vi "pressure_calcStress.vi"(9 "Pressure":dbl format="%#_13g", 10 "Angle":dbl, 11 "main_FGV_data":T1) -> (1 "PressCircOval":dbl, 2 "PressCirc":dbl, 3 "PressLong":dbl)   [LabVIEW 2016]
uses:
  MainFGV/main_FGV_data.ctl
  MainFGV/pipe_properties.ctl
  StressCalculations/point_data.ctl
  Ovalization/ovalization_data.ctl
  StressDist/StressDist_data.ctl
  StressDist/StressDist_single_data.ctl
  StressDist/Peirce/peirce_data.ctl
  pressure_data.ctl
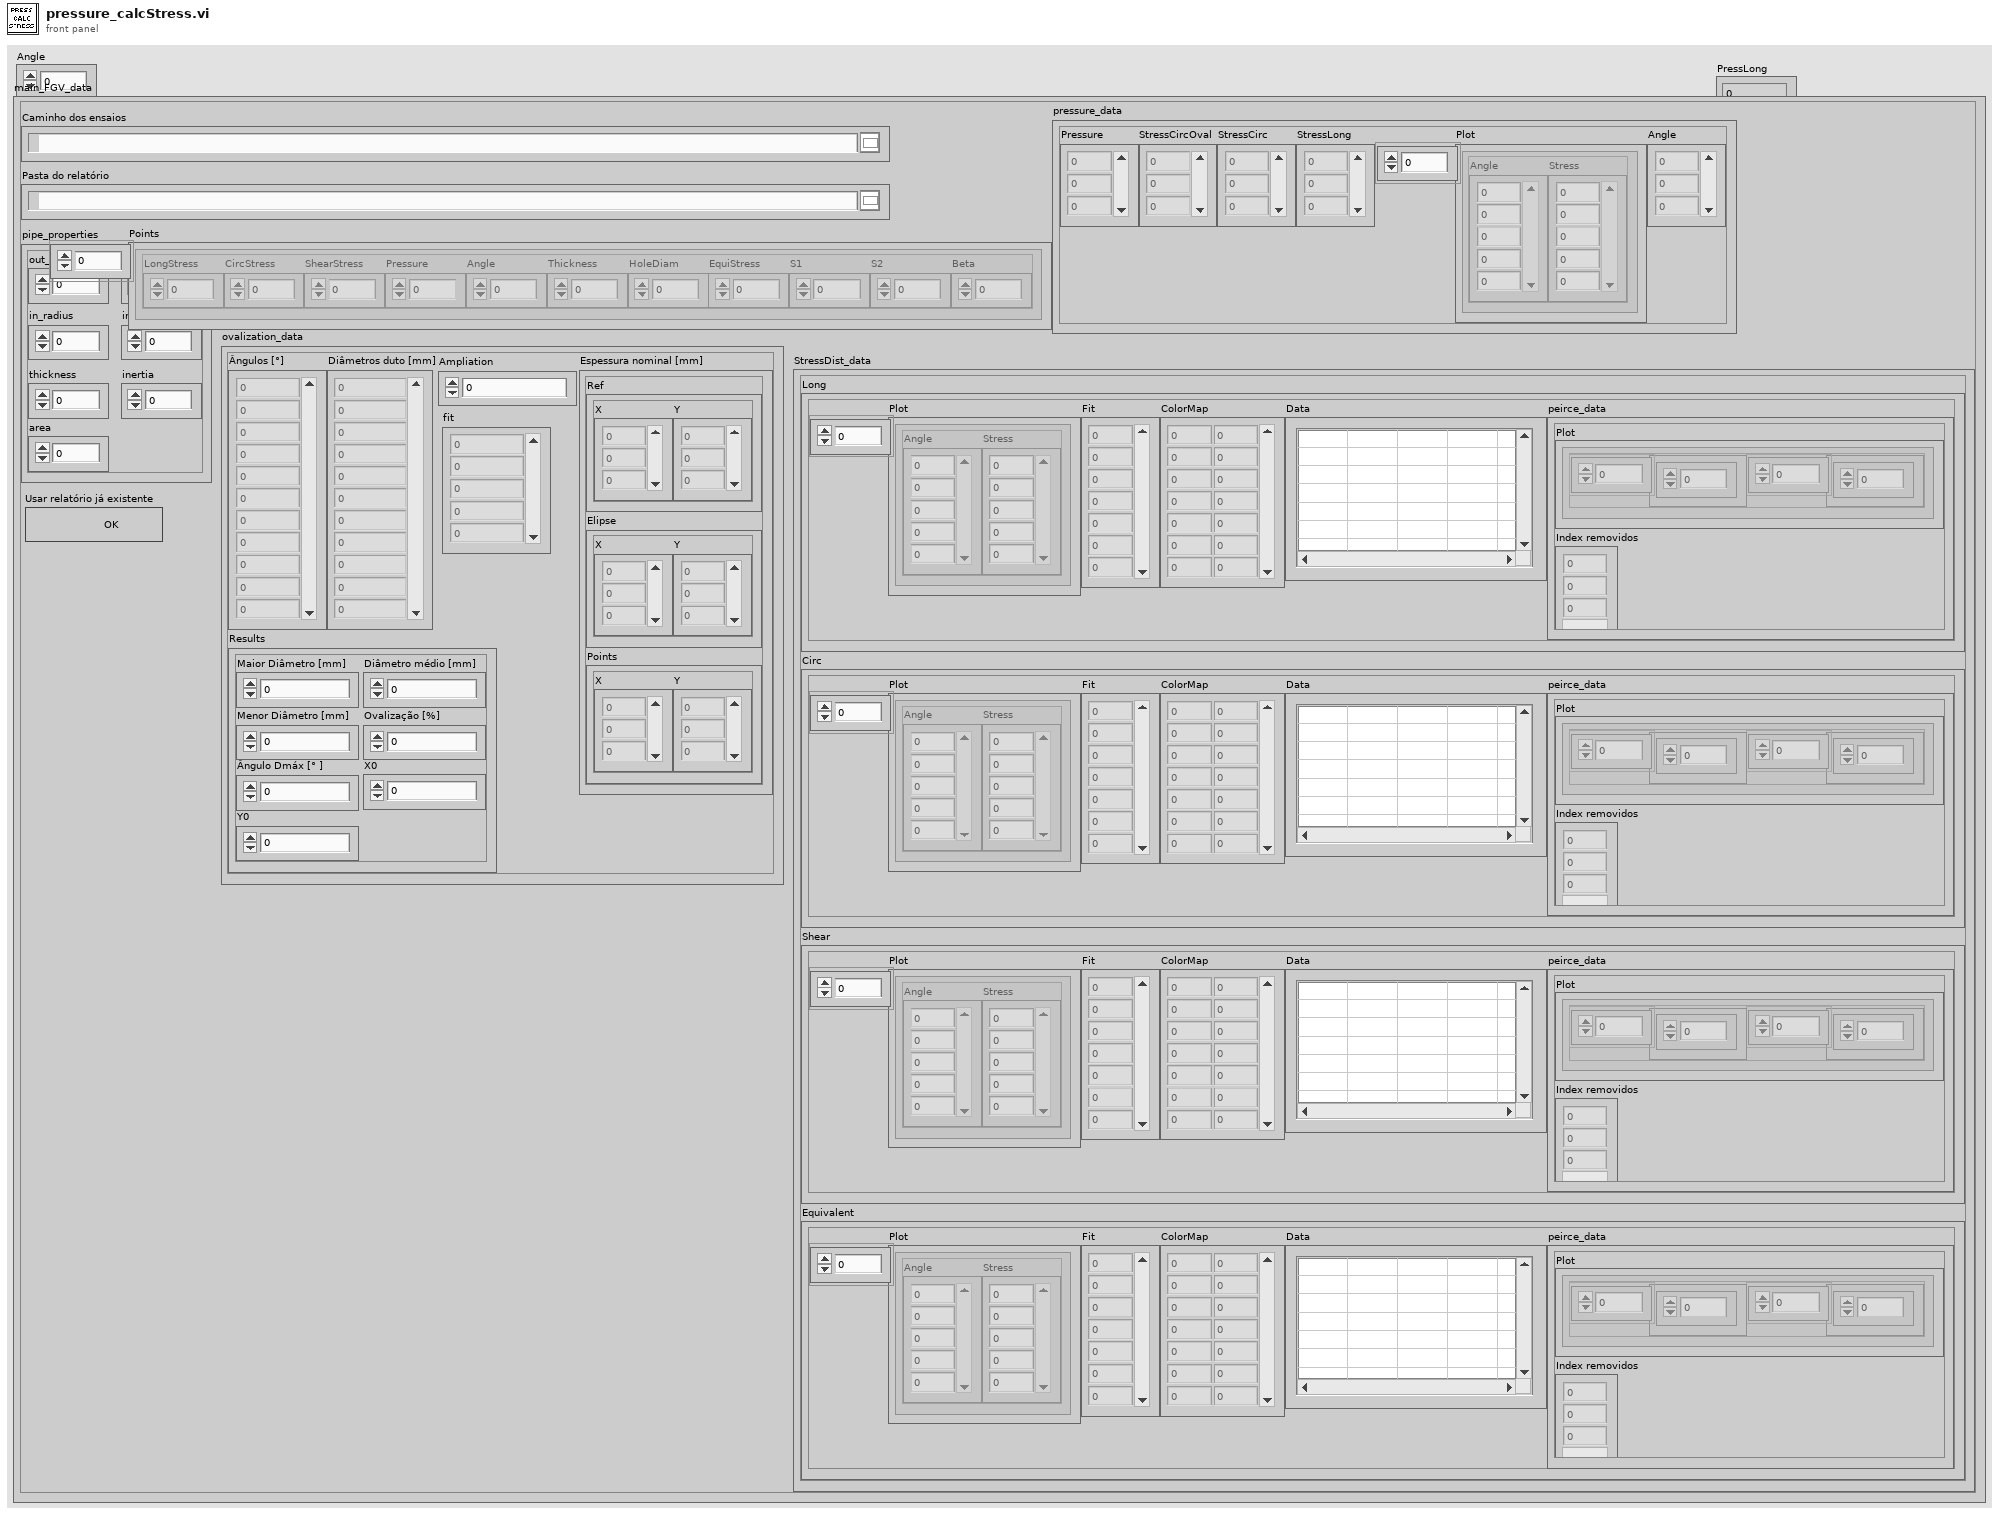
[diagram p1: front panel]
types:
  T1 = typedef "main_FGV_data.ctl" = cluster{"pipe_properties":T2, "DirPath":path, "DirReport":path, "Points":T3[], "ovalization_data":T4, "StressDist_data":T5, "pressure_data":T8, "Reload":bool}
  T2 = typedef "pipe_properties.ctl" = cluster{"out_radius":dbl, "in_radius":dbl, "out_diameter":dbl, "in_diameter":dbl, "thickness":dbl, "inertia":dbl, "area":dbl}
  T3 = typedef "point_data.ctl" = cluster{"LongStress":dbl, "CircStress":dbl, "ShearStress":dbl, "Pressure":dbl, "Angle":dbl, "Thickness":dbl, "HoleDiam":dbl, "EquiStress":dbl, "S1":dbl, "S2":dbl, "Beta":dbl}
  T4 = typedef "ovalization_data.ctl" = cluster{"AngOval":dbl[], "OvalDiam":dbl[], "Plots":cluster{"Ref":cluster{"X":dbl[], "Y":dbl[]}, "Elipse":cluster{"X":dbl[], "Y":dbl[]}, "Points":cluster{"X":dbl[], "Y":dbl[]}}, "Ampliation":dbl, "Results":cluster{"MD":dbl, "mD":dbl, "Dmed":dbl, "Oval":dbl, "ang":dbl, "X0":dbl, "Y0":dbl}, "fit":dbl[]}
  T5 = typedef "StressDist_data.ctl" = cluster{"Long":T6, "Circ":T6, "Shear":T6, "Equivalent":T6}
  T6 = typedef "StressDist_single_data.ctl" = cluster{"Plot":cluster{"Angle":dbl[], "Stress":dbl[]}[], "Fit":dbl[], "ColorMap":dbl[][], "Data":string[][], "peirce_data":T7}
  T7 = typedef "peirce_data.ctl" = cluster{"Plot":cluster{"Array":dbl[], "Array":dbl[]}[], "Index removidos":i32[]}
  T8 = typedef "pressure_data.ctl" = cluster{"Pressure":dbl[], "StressCircOval":dbl[], "StressCirc":dbl[], "StressLong":dbl[], "Plot":cluster{"Angle":dbl[], "Stress":dbl[]}[], "Angle":dbl[]}
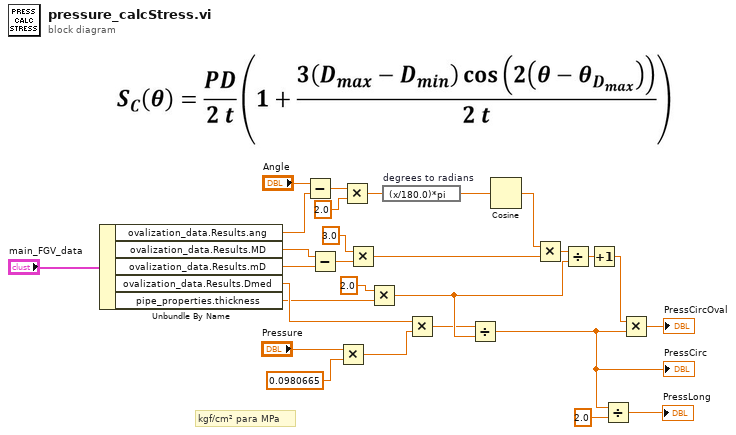
[diagram p0: block diagram]
diagram:
  # "kgf/cm² para MPa"
  n1 = Unbundle By Name("main_FGV_data") -> ("ovalization_data.Results.ang"=w15:dbl, "ovalization_data.Results.MD"=w10:dbl, "ovalization_data.Results.mD"=w11:dbl, "ovalization_data.Results.Dmed"=w23:dbl, "pipe_properties.thickness"=w20:dbl)
  n2 = Subtract(x="Angle", y=w15) -> (x-y=w13:dbl)
  n3 = Subtract(x=w10, y=w11) -> (x-y=w7:dbl)
  n4 = Multiply(x="Pressure", y=0.0980665) -> (x*y=w24:dbl)
  n5 = Multiply(x=w13, y=2.0) -> (x*y=w17:dbl)
  n6 = Multiply(x=3.0, y=w7) -> (x*y=w4:dbl)
  n7 = Multiply(x=2.0, y=w20) -> (x*y=w22:dbl)
  n8 = expression code="(x/180.0)*pi" "degrees to radians"(w17) -> (w18:dbl)
  n9 = Multiply(x=w23, y=w24) -> (x*y=w8:dbl)
  n10 = Divide(x=w8, y=w22) -> (x/y=w26:dbl)
  "PressCirc" <- w26
  n11 = Cosine(x=w18) -> (cos(x)=w5:dbl)
  n12 = Multiply(x=w5, y=w4) -> (x*y=w3:dbl)
  n13 = Divide(x=w3, y=w22) -> (x/y=w2:dbl)
  n14 = Increment(x=w2) -> (x+1=w1:dbl)
  n15 = Divide(x=w26, y=2.0) -> (x/y=→"PressLong":dbl)
  n16 = Multiply(x=w1, y=w26) -> (x*y=→"PressCircOval":dbl)
